vi "SET Enqueuers Array 2 Dispatch Message.vi"(8 "error in (no error)":errorcluster, 10 "Enqueuers Array":refnum<class "Message Enqueuer.lvclass">[](array[class]), 11 "Parent_Class in":refnum<class "Message_Distributor_Class.lvclass">) -> (0 "error out":errorcluster, 3 "Parent_Class out":refnum<class "Message_Distributor_Class.lvclass">)   [LabVIEW 2023, in "Actor_Message_Distributor.lvlib" / "Message_Distributor_Class.lvclass"]
uses:
  Message_Distributor_Class.lvclass
  <vilib>/ActorFramework/Message Enqueuer/Message Enqueuer.lvclass
  Message_Distributor_Class.lvclass/Message_Distributor_Class.ctl
panel:
  out "Parent Trigger Event Cluster.Data":string
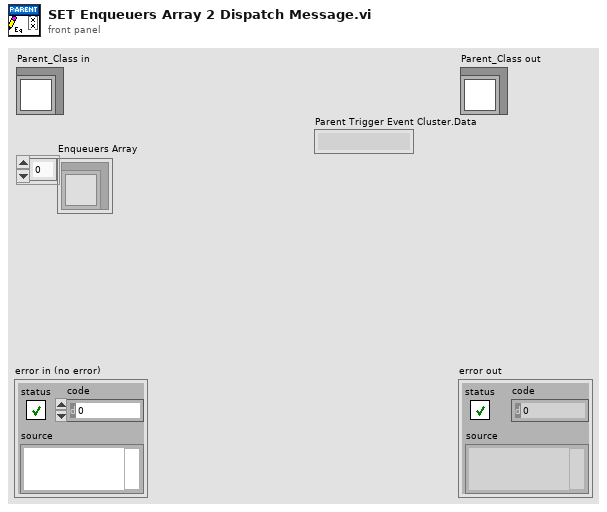
[diagram p1: front panel]
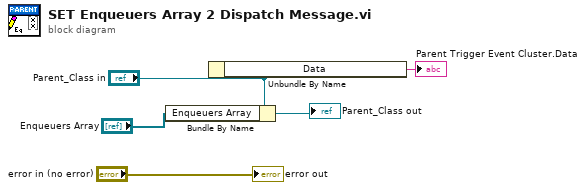
[diagram p0: block diagram]
diagram:
  n1 = Bundle By Name(cluster="Parent_Class in", "Enqueuers Array"="Enqueuers Array") -> (→"Parent_Class out":refnum<class "Message_Distributor_Class.lvclass">)
  n2 = Unbundle By Name("Parent_Class in") -> ("Data"=→"Parent Trigger Event Cluster.Data":string)
  "error out" <- "error in (no error)"
